vi "Fdx Get IRIG Time.vi"(8 "error in (no error)":errorcluster, 11 "InstrumentHandle_board in":u32) -> (0 "error out":errorcluster, 2 "Curent Irig Time":T1, 3 "InstrumentHandle_board out":u32)   [LabVIEW 2020, in "AIM664LV.lvlib"]
uses:
  AIM664LV.lvlib
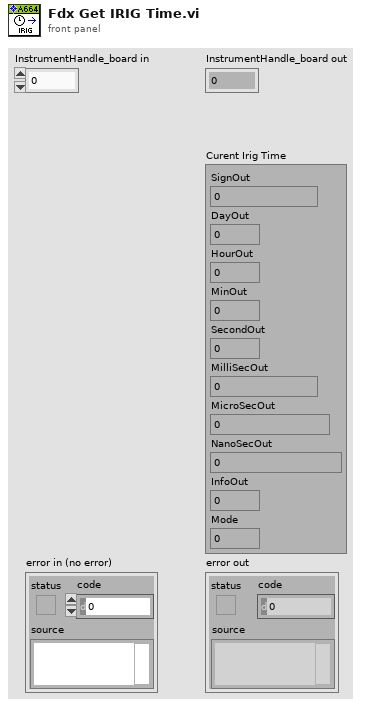
[diagram p1: front panel]
types:
  T1 = cluster{"SignOut":i32, "DayOut":u32, "HourOut":u32, "MinOut":u32, "SecondOut":u32, "MilliSecOut":u32, "MicroSecOut":u32, "NanoSecOut":u32, "InfoOut":u32, "Mode":u32}
  T2 = cluster{"Control":u32, "SignIn":i32, "DayIn":u32, "HourIn":u32, "MinIn":u32, "SecondIn":u32, "MilliSecIn":u32, "MicroSecIn":u32, "NanoSecIn":u32, "InfoIn":u32}
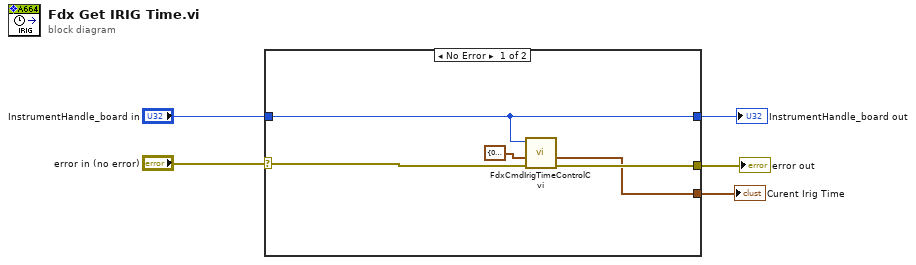
[diagram p0: block diagram]
diagram:
  n1 = case shown="No Error" "error in (no error)" {
    selector: "error in (no error)" -> [w9 w12]
    tunnel: [w8 w12] -> w4
    tunnel: [w6 w11] -> w2
    tunnel: "InstrumentHandle_board in" -> [w6 w11]
    tunnel: [w7 _] -> w1
    frame No Error {
      n2 = call "FdxCmdIrigTimeControlCvi.vi"("error in"=w9, "Irig In"=T2 {"Control"=0, "SignIn"=0, "DayIn"=0, "HourIn"=0, "MinIn"=0, "SecondIn"=0, "MilliSecIn"=0, "MicroSecIn"=0, "NanoSecIn"=0, "InfoIn"=0}, "InstrumentHandle_board in"=w6) -> ("error out"=w8:errorcluster, "Irig Out"=w7:T1)  [unwired: 6 in, 1 out]
    }
    frame Error {
    }
  }
  "error out" <- w4
  "InstrumentHandle_board out" <- w2
  "Curent Irig Time" <- w1
